vi "SPIM_LIVE.vi"() -> ()   [LabVIEW 2012]
panel:
  in  "Frames":i32=100
  out "Frames Recorded":i32=100
  in  "DCIMG Path":path=path "H:/test3.ps"
  out "Display":T1(plugin-control)
  out "Camera Serial":string="S/N: 730852"
  out "Camera Version":string="2.50.A"
  out "Camera Model":string="C11440-22C"
  out "SMD":dbl=2.0
  in  "Scan Mode":dbl=2.0 min=1.0 max=2.0 step=1.0
  in  "Exposure":dbl=0.00999771 min=0.0010036691729323308 max=10.0 step=1e-08
  out "EXP":dbl=0.00999771
  out "SVW":i32=2048
  out "SHW":i32=2048
  out "SVO":i32
  out "SHO":i32
  in  "V Width":i32=2048 min=1 max=512 step=1
  in  "V Offset":i32 min=0 max=0 step=1
  in  "H Width":i32=2048 min=1 max=512 step=1
  in  "H Offset":i32 min=0 max=0 step=1
  in  "Binning":u16(ring)=4 items=["1x1"=1, "2x2"=2, "4x4"=4]
  out "Elapsed Time":u32=7532
  out "Total Frames":i32=633
  in  "Display":bool=TRUE
  out "Frames Per Second":dbl=100.0
  out "error out":errorcluster
  in  "stop":bool
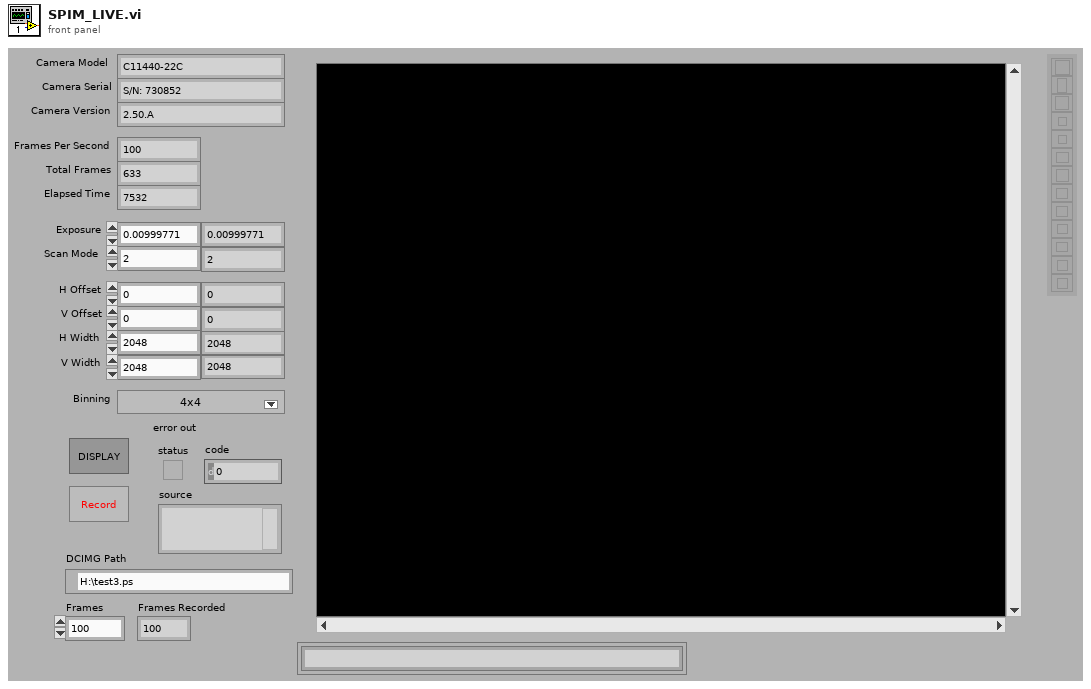
[diagram p1: front panel]
types:
  T1 = typedef "IMAQ Image.ctl" = refnum<image>
  T2 = typedef "Image Type" = u32
  T3 = cluster{"Value":i32, "Minimum":i32, "Maximum":i32, "Increment":i32}
  T4 = cluster{"width":u32, "height":u32, "datatype":u32}
  T5 = cluster{"H Offset":i32, "V Offset":i32, "H Width":i32, "V Width":i32}
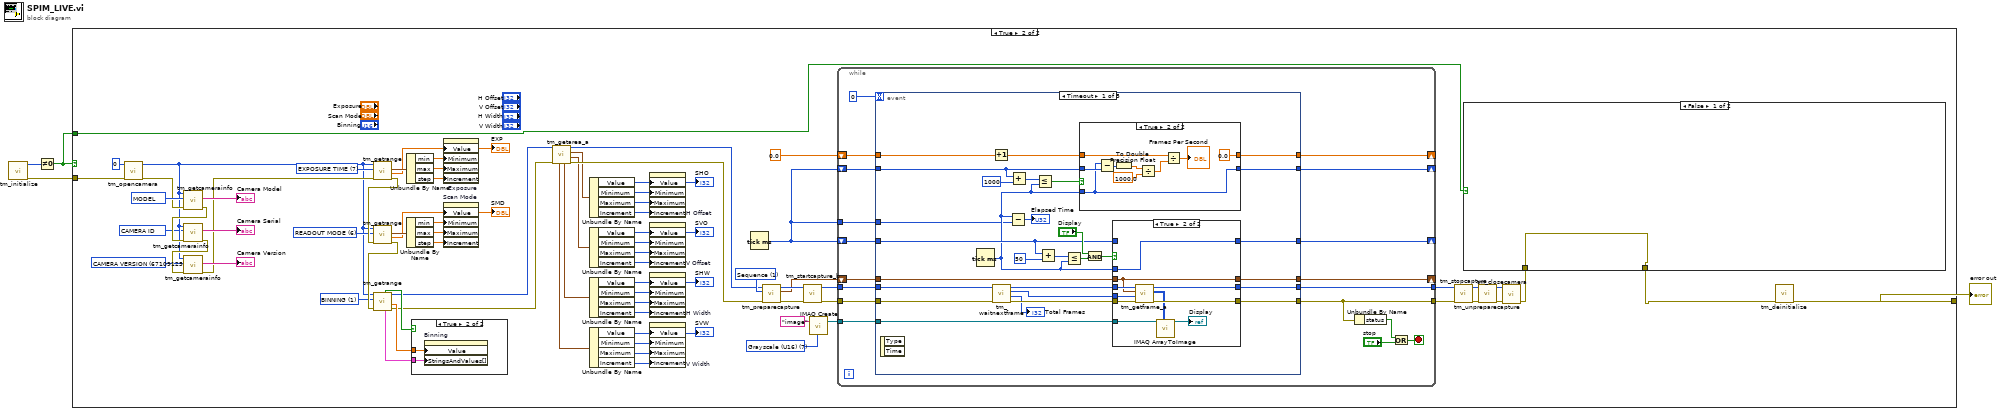
[diagram p0: block diagram]
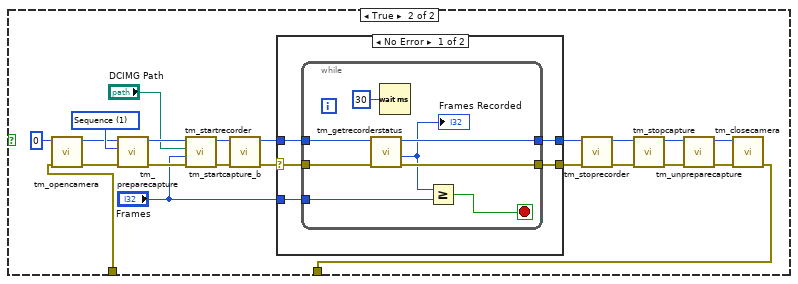
[diagram p3: hidden frame]
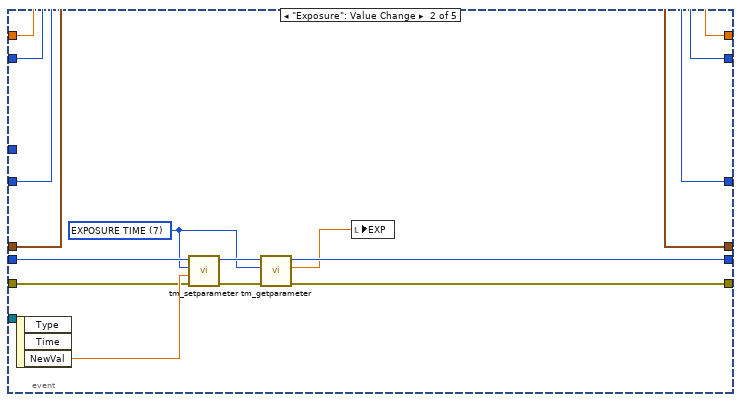
[diagram p8: hidden frame]
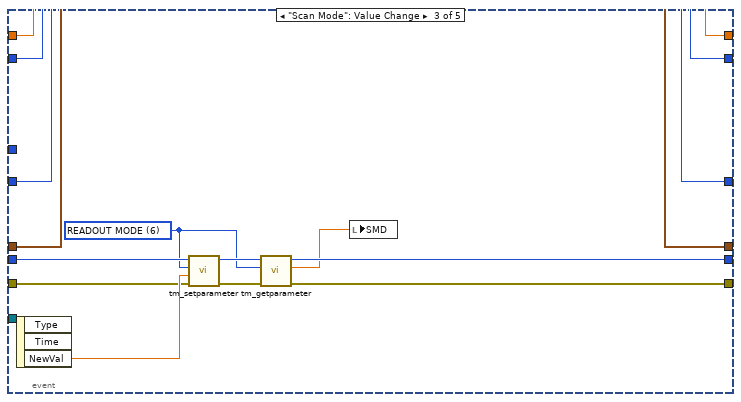
[diagram p9: hidden frame]
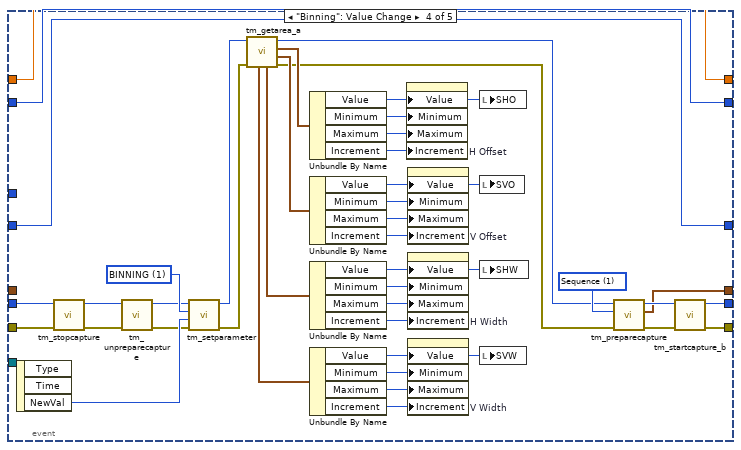
[diagram p10: hidden frame]
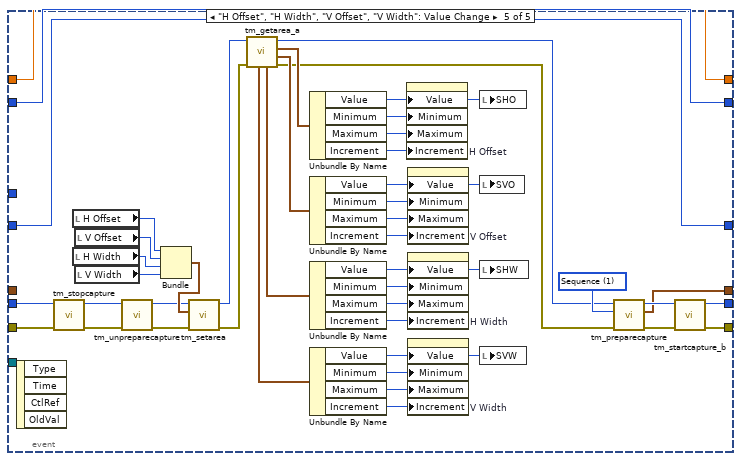
[diagram p11: hidden frame]
diagram:
  n1 = call <userlib>:"tm_initialize.vi"() -> ("error out"=w3:errorcluster, "Number Of Cameras"=w2:u32)  [unwired: 10 in]
  n2 = Not Equal To 0?(x=w2) -> (x != 0?=w1:bool)
  n3 = case shown="True" w1 {
    tunnel: [w5 w79] -> w4
    tunnel: w3 -> [w5 w81]
    tunnel: w1 -> [_ w8]
    frame False {
    }
    frame True {
      w9 = T2 7 items=["Grayscale (U8)", "Grayscale (I16)", "Grayscale (SGL)", "Complex (CSG)", "RGB (U32)", "HSL (U32)", "RGB (U64)", "Grayscale (U16)"] ("Image Type")
      w23 = u32 67109122 items=["BUS"=67109121, "CAMERA ID"=67109122, "VENDOR"=67109123, "MODEL"=67109124, "CAMERA VERSION"=67109125, "DRIVER VERSION"=67109126, "MODULE VERSIOIN"=67109127, "DCAMAPI VERSION"=67109128] ("Info ID")
      w30 = u32 67109125 items=["BUS"=67109121, "CAMERA"=67109122, "VENDOR"=67109123, "MODEL"=67109124, "CAMERA VERSION"=67109125, "DRIVER VERSION"=67109126, "MODULE VERSIOIN"=67109127, "DCAMAPI VERSION"=67109128] ("Info ID")
      w33 = u32 67109124 items=["BUS"=67109121, "CAMERA"=67109122, "VENDOR"=67109123, "MODEL"=67109124, "CAMERA VERSION"=67109125, "DRIVER VERSION"=67109126, "MODULE VERSIOIN"=67109127, "DCAMAPI VERSION"=67109128] ("Info ID")
      w65 = 1 items=["BINNING"=1, "BITS PER CHANNEL"=2, "ACTIVE VIEW INDEX"=3, "CCD MODE"=4, "SENSOR MODE"=5, "READOUT MODE"=6, "EXPOSURE TIME"=7, "CONTRAST GAIN"=8, "CONTRAST OFFSET"=9, "LIGHT MODE"=10, "SENSITIVITY"=11, "WHITE BALANCE"=12, "PHOTON IMAGING MODE"=13, "HIGH DYNAMIC RANGE MODE"=14, "TRIGGER SOURCE"=15, "TRIGGER ACTIVE"=16, "TRIGGER MODE"=17, "TRIGGER POLARITY"=18, "TRIGGER GLOBAL EXPOSURE"=19, "FIRST TRIGGER BEHAVIOR"=20, "TRIGGER TIMES"=21, "OUTPUT TRIGGER POLARITY"=22, "OUTPUT TRIGGER DELAY"=23, "OUTPUT TRIGGER PERIOD"=24, "TEMPERATURE"=25, "TEMPERATURE TARGET"=26, "SENSOR COOLER FAN"=27, "MECHANICAL SHUTTER"=28, "BACK FOCUS POSITION"=29, "FRAMEBUNDLE MODE"=30, "FRAMEBUNDLE NUMBER"=31] ("Parameter")
      w67 = 6 items=["BINNING"=1, "BITS PER CHANNEL"=2, "ACTIVE VIEW INDEX"=3, "CCD MODE"=4, "SENSOR MODE"=5, "READOUT MODE"=6, "EXPOSURE TIME"=7, "CONTRAST GAIN"=8, "CONTRAST OFFSET"=9, "LIGHT MODE"=10, "SENSITIVITY"=11, "WHITE BALANCE"=12, "PHOTON IMAGING MODE"=13, "HIGH DYNAMIC RANGE MODE"=14, "TRIGGER SOURCE"=15, "TRIGGER ACTIVE"=16, "TRIGGER MODE"=17, "TRIGGER POLARITY"=18, "TRIGGER GLOBAL EXPOSURE"=19, "FIRST TRIGGER BEHAVIOR"=20, "TRIGGER TIMES"=21, "OUTPUT TRIGGER POLARITY"=22, "OUTPUT TRIGGER DELAY"=23, "OUTPUT TRIGGER PERIOD"=24, "TEMPERATURE"=25, "TEMPERATURE TARGET"=26, "SENSOR COOLER FAN"=27, "MECHANICAL SHUTTER"=28, "BACK FOCUS POSITION"=29, "FRAMEBUNDLE MODE"=30, "FRAMEBUNDLE NUMBER"=31] ("Parameter")
      w70 = 7 items=["BINNING"=1, "BITS PER CHANNEL"=2, "ACTIVE VIEW INDEX"=3, "CCD MODE"=4, "SENSOR MODE"=5, "READOUT MODE"=6, "EXPOSURE TIME"=7, "CONTRAST GAIN"=8, "CONTRAST OFFSET"=9, "LIGHT MODE"=10, "SENSITIVITY"=11, "WHITE BALANCE"=12, "PHOTON IMAGING MODE"=13, "HIGH DYNAMIC RANGE MODE"=14, "TRIGGER SOURCE"=15, "TRIGGER ACTIVE"=16, "TRIGGER MODE"=17, "TRIGGER POLARITY"=18, "TRIGGER GLOBAL EXPOSURE"=19, "FIRST TRIGGER BEHAVIOR"=20, "TRIGGER TIMES"=21, "OUTPUT TRIGGER POLARITY"=22, "OUTPUT TRIGGER DELAY"=23, "OUTPUT TRIGGER PERIOD"=24, "TEMPERATURE"=25, "TEMPERATURE TARGET"=26, "SENSOR COOLER FAN"=27, "MECHANICAL SHUTTER"=28, "BACK FOCUS POSITION"=29, "FRAMEBUNDLE MODE"=30, "FRAMEBUNDLE NUMBER"=31] ("Parameter")
      w77 = 1 items=["Snap", "Sequence"] ("Capture mode")
      n4 = call <userlib>:"tm_opencamera.vi"("error in (no error)"=w81, "Camera Index"=u32 0) -> ("error out"=w26:errorcluster, "Handle out"=w24:u32)  [unwired: 8 in]
      n5 = call <userlib>:"tm_getcamerainfo.vi"("error in (no error)"=w26, "Info ID"=w33, "Handle in"=w24) -> ("error out"=w32:errorcluster, "String"=→"Camera Model":string)  [unwired: 6 in, 1 out]
      n6 = call <userlib>:"tm_getcamerainfo.vi"("error in (no error)"=w32, "Info ID"=w23, "Handle in"=w24) -> ("error out"=w31:errorcluster, "String"=→"Camera Serial":string)  [unwired: 6 in, 1 out]
      n7 = call <userlib>:"tm_getcamerainfo.vi"("error in (no error)"=w31, "Info ID"=w30, "Handle in"=w24) -> ("error out"=w25:errorcluster, "String"=→"Camera Version":string)  [unwired: 6 in, 1 out]
      n8 = call <userlib>:"tm_getrange.vi"("error in (no error)"=w25, "Parameter"=w70, "Handle in"=w24) -> ("error out"=w68:errorcluster, "default"=w61:dbl, "Range"=w69:cluster{"min":dbl, "max":dbl, "step":dbl})  [unwired: 2 in, 4 out]
      "EXP" <- w61
      n9 = call <userlib>:"tm_getrange.vi"("error in (no error)"=w68, "Parameter"=w67, "Handle in"=w24) -> ("error out"=w66:errorcluster, "default"=w56:dbl, "Range"=w60:cluster{"min":dbl, "max":dbl, "step":dbl})  [unwired: 2 in, 4 out]
      "SMD" <- w56
      n10 = call <userlib>:"tm_getrange.vi"("error in (no error)"=w66, "Parameter"=w65, "Handle in"=w24) -> ("error out"=w51:errorcluster, "default"=w53:dbl, "Handle out"=w52:u32, "Value Names"=w54:cluster{"Name":string, "Value":dbl}[], "Writable"=w55:bool)  [unwired: 2 in, 2 out]
      n11 = Unbundle By Name(w69) -> ("min"=w64:dbl, "max"=w63:dbl, "step"=w62:dbl)
      n12 = Unbundle By Name(w60) -> ("min"=w59:dbl, "max"=w58:dbl, "step"=w57:dbl)
      n13 = case shown="True" w55 {
        tunnel: w54 -> [_ w121]
        tunnel: w53 -> [_ w120]
        frame False {
        }
        frame True {
          n14 = property on="Binning" class="Ring (strict)"("Value"=w120, "StringsAndValues[]"=w121) -> ()  [unwired: 2 in, 2 out]
        }
      }
      n15 = property on="Exposure" class="DigNum (strict)"("Value"=w61, "Minimum"=w64, "Maximum"=w63, "Increment"=w62) -> ()  [unwired: 2 in, 2 out]
      n16 = property on="Scan Mode" class="DigNum (strict)"("Value"=w56, "Minimum"=w59, "Maximum"=w58, "Increment"=w57) -> ()  [unwired: 2 in, 2 out]
      n17 = call <userlib>:"tm_getarea_a.vi"("error in (no error)"=w51, "Handle in"=w52) -> ("error out"=w49:errorcluster, "V Offset"=w48:T3, "H Offset"=w16:T3, "Handle out"=w50:u32, "H Width"=w47:T3, "V Width"=w46:T3)  [unwired: 4 in]
      n18 = Unbundle By Name(w16) -> ("Value"=w15:i32, "Minimum"=w14:i32, "Maximum"=w13:i32, "Increment"=w12:i32)
      "SHO" <- w15
      n19 = Unbundle By Name(w48) -> ("Value"=w36:i32, "Minimum"=w45:i32, "Maximum"=w44:i32, "Increment"=w43:i32)
      "SVO" <- w36
      n20 = Unbundle By Name(w47) -> ("Value"=w35:i32, "Minimum"=w42:i32, "Maximum"=w41:i32, "Increment"=w40:i32)
      "SHW" <- w35
      n21 = Unbundle By Name(w46) -> ("Value"=w34:i32, "Minimum"=w39:i32, "Maximum"=w38:i32, "Increment"=w37:i32)
      "SVW" <- w34
      n22 = property on="H Offset" class="DigNum (strict)"("Value"=w15, "Minimum"=w14, "Maximum"=w13, "Increment"=w12) -> ()  [unwired: 2 in, 2 out]
      n23 = property on="V Offset" class="DigNum (strict)"("Value"=w36, "Minimum"=w45, "Maximum"=w44, "Increment"=w43) -> ()  [unwired: 2 in, 2 out]
      n24 = property on="H Width" class="DigNum (strict)"("Value"=w35, "Minimum"=w42, "Maximum"=w41, "Increment"=w40) -> ()  [unwired: 2 in, 2 out]
      n25 = property on="V Width" class="DigNum (strict)"("Value"=w34, "Minimum"=w39, "Maximum"=w38, "Increment"=w37) -> ()  [unwired: 2 in, 2 out]
      n26 = Tick Count (ms)() -> (millisecond timer value=w71:u32)
      n27 = call <userlib>:"tm_preparecapture.vi"("error in (no error)"=w49, "Capture mode"=w77, "Handle in"=w50) -> ("error out"=w75:errorcluster, "Buffer"=w72:T4, "Handle out"=w76:u32)  [unwired: 5 in, 1 out]
      n28 = call <userlib>:"tm_startcapture_b.vi"("error in (no error)"=w75, "Handle in"=w76) -> ("error out"=w74:errorcluster, "Handle out"=w73:u32)  [unwired: 8 in]
      n29 = call "IMAQ Create"("Image Name"="image", "Image Type"=w9) -> ("New Image"=w10:T1)  [unwired: 3 in, 1 out]
      n30 = while {
        tunnel: w74 -> [w127]
        tunnel: [w125] -> w22
        tunnel: [w124] -> w21
        shift-right: [w134] -> _
        shift-left: w71 -> [w132]
        shift-right: [w135] -> _
        shift-left: 0.0 -> [w133]
        shift-right: [w126] -> _
        shift-left: w71 -> [w130]
        tunnel: w73 -> [w128]
        tunnel: w71 -> [w131]
        shift-right: [w123] -> _
        shift-left: w72 -> [w129]
        tunnel: w10 -> [w122]
        stop <- w137 stop-if-true
        n31 = event shown="[0] Timeout" {
          selector: _ -> [_ _ _ _ _]
          dyn-events: _ -> [_ _ _ _ _]
          timeout: 0 -> [_ _ _ _ _]
          tunnel: [w148 w203 w216 w250 w296] -> w135
          tunnel: [w147 w204 w217 w251 w297] -> w134
          tunnel: w133 -> [w149 w203 w216 w250 w296]
          tunnel: w132 -> [w151 w204 w217 w251 w297]
          tunnel: w131 -> [w143 _ _ _ _]
          tunnel: w130 -> [w152 w206 w219 w260 w304]
          tunnel: w129 -> [w142 w195 w208 _ _]
          tunnel: w128 -> [w154 w201 w214 w225 w266]
          tunnel: w127 -> [w153 w202 w215 w224 w265]
          tunnel: [w146 w206 w219 w260 w304] -> w126
          tunnel: [w145 w197 w210 w254 w299] -> w125
          tunnel: [w144 w196 w209 w255 w300] -> w124
          tunnel: [w141 w195 w208 w253 w298] -> w123
          tunnel: w122 -> [w140 _ _ _ _]
          event Timeout {
            n32 = event-data() -> ()  [unwired: 1 in, 2 out]
            n33 = Tick Count (ms)() -> (millisecond timer value=w150:u32)
            n34 = Increment(x=w149) -> (x+1=w165:dbl)
            n35 = call <userlib>:"tm_waitnextframe.vi"("error in (no error)"=w153, "Handle in"=w154) -> ("error out"=w159:errorcluster, "Frame Count"=→"Total Frames":i32, "Frame Index"=w158:i32, "Handle out"=w160:u32)  [unwired: 6 in]
            n36 = Subtract(x=w150, y=w143) -> (x-y=→"Elapsed Time":u32)
            n37 = Add(x=w151, y=u32 1000) -> (x+y=w168:u32)
            n38 = Less Or Equal?(x=w168, y=w150) -> (x <= y?=w167:bool)
            n39 = Add(x=w152, y=u32 50) -> (x+y=w164:u32)
            n40 = Less Or Equal?(x=w164, y=w150) -> (x <= y?=w162:bool)
            n41 = case shown="True" w167 {
              tunnel: w151 -> [w184 w187]
              tunnel: [w184 w185] -> w147
              tunnel: w165 -> [w183 w191]
              tunnel: w150 -> [_ w185]
              tunnel: [w183 0.0] -> w148
              frame False {
              }
              frame True {
                n42 = Subtract(x=w185, y=w187) -> (x-y=w186:u32)
                n43 = To Double Precision Float(number=w186) -> (double precision float=w193:dbl)
                n44 = Divide(x=w193, y=1000.0) -> (x/y=w190:dbl)
                n45 = Divide(x=w191, y=w190) -> (x/y=→"Frames Per Second":dbl)
              }
            }
            n46 = And(x="Display", y=w162) -> (x .and. y?=w157:bool)
            n47 = case shown="True" w157 {
              tunnel: w152 -> [w172 _]
              tunnel: w150 -> [_ w182]
              tunnel: [w172 w182] -> w146
              tunnel: w160 -> [w171 w181]
              tunnel: w142 -> [w169 w176]
              tunnel: w159 -> [w170 w180]
              tunnel: [w171 w179] -> w145
              tunnel: [w170 w178] -> w144
              tunnel: w158 -> [_ w177]
              tunnel: [w169 w176] -> w141
              tunnel: w140 -> [_ w174]
              frame False {
              }
              frame True {
                n48 = call <userlib>:"tm_getframe_a.vi"("error in (no error)"=w180, "Frame Index"=w177, "Buffer"=w176, "Handle in"=w181) -> ("error out"=w178:errorcluster, "Data 16"=w175:u16[][], "Handle out"=w179:u32)  [unwired: 3 in, 2 out]
                n49 = call "IMAQ ArrayToImage"("Image Pixels (U16)"=w175, "Image"=w174) -> ("Image Out"=→"Display":T1)  [unwired: 8 in, 1 out]
              }
            }
          }
          event "Exposure": Value Change {
            w198 = 7 items=["BINNING"=1, "BITS PER CHANNEL"=2, "ACTIVE VIEW INDEX"=3, "CCD MODE"=4, "SENSOR MODE"=5, "READOUT MODE"=6, "EXPOSURE TIME"=7, "CONTRAST GAIN"=8, "CONTRAST OFFSET"=9, "LIGHT MODE"=10, "SENSITIVITY"=11, "WHITE BALANCE"=12, "PHOTON IMAGING MODE"=13, "HIGH DYNAMIC RANGE MODE"=14, "TRIGGER SOURCE"=15, "TRIGGER ACTIVE"=16, "TRIGGER MODE"=17, "TRIGGER POLARITY"=18, "TRIGGER GLOBAL EXPOSURE"=19, "FIRST TRIGGER BEHAVIOR"=20, "TRIGGER TIMES"=21, "OUTPUT TRIGGER POLARITY"=22, "OUTPUT TRIGGER DELAY"=23, "OUTPUT TRIGGER PERIOD"=24, "TEMPERATURE"=25, "TEMPERATURE TARGET"=26, "SENSOR COOLER FAN"=27, "MECHANICAL SHUTTER"=28, "BACK FOCUS POSITION"=29, "FRAMEBUNDLE MODE"=30, "FRAMEBUNDLE NUMBER"=31] ("Parameter")
            n50 = event-data() -> ("NewVal"=w205:dbl)  [unwired: 1 in, 2 out]
            n51 = call <userlib>:"tm_setparameter.vi"("error in (no error)"=w202, "Value in"=w205, "Parameter"=w198, "Handle in"=w201) -> ("error out"=w200:errorcluster, "Handle out"=w199:u32)  [unwired: 6 in]
            n52 = call <userlib>:"tm_getparameter.vi"("error in (no error)"=w200, "Parameter"=w198, "Handle in"=w199) -> ("error out"=w196:errorcluster, "Value out"=w194:dbl, "Handle out"=w197:u32)  [unwired: 6 in]
            n53 = local write "EXP"(w194) -> ()
          }
          event "Scan Mode": Value Change {
            w211 = 6 items=["BINNING"=1, "BITS PER CHANNEL"=2, "ACTIVE VIEW INDEX"=3, "CCD MODE"=4, "SENSOR MODE"=5, "READOUT MODE"=6, "EXPOSURE TIME"=7, "CONTRAST GAIN"=8, "CONTRAST OFFSET"=9, "LIGHT MODE"=10, "SENSITIVITY"=11, "WHITE BALANCE"=12, "PHOTON IMAGING MODE"=13, "HIGH DYNAMIC RANGE MODE"=14, "TRIGGER SOURCE"=15, "TRIGGER ACTIVE"=16, "TRIGGER MODE"=17, "TRIGGER POLARITY"=18, "TRIGGER GLOBAL EXPOSURE"=19, "FIRST TRIGGER BEHAVIOR"=20, "TRIGGER TIMES"=21, "OUTPUT TRIGGER POLARITY"=22, "OUTPUT TRIGGER DELAY"=23, "OUTPUT TRIGGER PERIOD"=24, "TEMPERATURE"=25, "TEMPERATURE TARGET"=26, "SENSOR COOLER FAN"=27, "MECHANICAL SHUTTER"=28, "BACK FOCUS POSITION"=29, "FRAMEBUNDLE MODE"=30, "FRAMEBUNDLE NUMBER"=31] ("Parameter")
            n54 = event-data() -> ("NewVal"=w218:dbl)  [unwired: 1 in, 2 out]
            n55 = call <userlib>:"tm_setparameter.vi"("error in (no error)"=w215, "Value in"=w218, "Parameter"=w211, "Handle in"=w214) -> ("error out"=w213:errorcluster, "Handle out"=w212:u32)  [unwired: 6 in]
            n56 = call <userlib>:"tm_getparameter.vi"("error in (no error)"=w213, "Parameter"=w211, "Handle in"=w212) -> ("error out"=w209:errorcluster, "Value out"=w207:dbl, "Handle out"=w210:u32)  [unwired: 6 in]
            n57 = local write "SMD"(w207) -> ()
          }
          event "Binning": Value Change {
            w258 = 1 items=["Snap", "Sequence"] ("Capture mode")
            w259 = 1 items=["BINNING"=1, "BITS PER CHANNEL"=2, "ACTIVE VIEW INDEX"=3, "CCD MODE"=4, "SENSOR MODE"=5, "READOUT MODE"=6, "EXPOSURE TIME"=7, "CONTRAST GAIN"=8, "CONTRAST OFFSET"=9, "LIGHT MODE"=10, "SENSITIVITY"=11, "WHITE BALANCE"=12, "PHOTON IMAGING MODE"=13, "HIGH DYNAMIC RANGE MODE"=14, "TRIGGER SOURCE"=15, "TRIGGER ACTIVE"=16, "TRIGGER MODE"=17, "TRIGGER POLARITY"=18, "TRIGGER GLOBAL EXPOSURE"=19, "FIRST TRIGGER BEHAVIOR"=20, "TRIGGER TIMES"=21, "OUTPUT TRIGGER POLARITY"=22, "OUTPUT TRIGGER DELAY"=23, "OUTPUT TRIGGER PERIOD"=24, "TEMPERATURE"=25, "TEMPERATURE TARGET"=26, "SENSOR COOLER FAN"=27, "MECHANICAL SHUTTER"=28, "BACK FOCUS POSITION"=29, "FRAMEBUNDLE MODE"=30, "FRAMEBUNDLE NUMBER"=31] ("Parameter")
            n58 = event-data() -> ("NewVal"=w252:u16)  [unwired: 1 in, 2 out]
            n59 = call <userlib>:"tm_stopcapture.vi"("error in (no error)"=w224, "Handle in"=w225) -> ("error out"=w220:errorcluster, "Handle out"=w223:u32)  [unwired: 8 in]
            n60 = call <userlib>:"tm_unpreparecapture.vi"("error in (no error)"=w220, "Handle in"=w223) -> ("error out"=w221:errorcluster, "Handle out"=w222:u32)  [unwired: 8 in]
            n61 = call <userlib>:"tm_setparameter.vi"("error in (no error)"=w221, "Value in"=w252, "Parameter"=w259, "Handle in"=w222) -> ("error out"=w244:errorcluster, "Handle out"=w245:u32)  [unwired: 6 in]
            n62 = call <userlib>:"tm_getarea_a.vi"("error in (no error)"=w244, "Handle in"=w245) -> ("error out"=w243:errorcluster, "V Offset"=w247:T3, "H Offset"=w246:T3, "Handle out"=w242:u32, "H Width"=w248:T3, "V Width"=w249:T3)  [unwired: 4 in]
            n63 = Unbundle By Name(w246) -> ("Value"=w238:i32, "Minimum"=w241:i32, "Maximum"=w240:i32, "Increment"=w239:i32)
            n64 = Unbundle By Name(w247) -> ("Value"=w228:i32, "Minimum"=w237:i32, "Maximum"=w236:i32, "Increment"=w235:i32)
            n65 = Unbundle By Name(w248) -> ("Value"=w227:i32, "Minimum"=w234:i32, "Maximum"=w233:i32, "Increment"=w232:i32)
            n66 = Unbundle By Name(w249) -> ("Value"=w226:i32, "Minimum"=w231:i32, "Maximum"=w230:i32, "Increment"=w229:i32)
            n67 = property on="H Offset" class="DigNum (strict)"("Value"=w238, "Minimum"=w241, "Maximum"=w240, "Increment"=w239) -> ()  [unwired: 2 in, 2 out]
            n68 = property on="V Offset" class="DigNum (strict)"("Value"=w228, "Minimum"=w237, "Maximum"=w236, "Increment"=w235) -> ()  [unwired: 2 in, 2 out]
            n69 = property on="H Width" class="DigNum (strict)"("Value"=w227, "Minimum"=w234, "Maximum"=w233, "Increment"=w232) -> ()  [unwired: 2 in, 2 out]
            n70 = property on="V Width" class="DigNum (strict)"("Value"=w226, "Minimum"=w231, "Maximum"=w230, "Increment"=w229) -> ()  [unwired: 2 in, 2 out]
            n71 = local write "SHO"(w238) -> ()
            n72 = local write "SVO"(w228) -> ()
            n73 = local write "SHW"(w227) -> ()
            n74 = local write "SVW"(w226) -> ()
            n75 = call <userlib>:"tm_preparecapture.vi"("error in (no error)"=w243, "Capture mode"=w258, "Handle in"=w242) -> ("error out"=w256:errorcluster, "Buffer"=w253:T4, "Handle out"=w257:u32)  [unwired: 5 in, 1 out]
            n76 = call <userlib>:"tm_startcapture_b.vi"("error in (no error)"=w256, "Handle in"=w257) -> ("error out"=w255:errorcluster, "Handle out"=w254:u32)  [unwired: 8 in]
          }
          event "H Offset", "H Width", "V Offset", "V Width": Value Change {
            w303 = 1 items=["Snap", "Sequence"] ("Capture mode")
            n77 = event-data() -> ()  [unwired: 1 in, 4 out]
            n78 = call <userlib>:"tm_stopcapture.vi"("error in (no error)"=w265, "Handle in"=w266) -> ("error out"=w263:errorcluster, "Handle out"=w264:u32)  [unwired: 8 in]
            n79 = local read "H Offset"() -> (w269:i32)
            n80 = local read "H Width"() -> (w270:i32)
            n81 = local read "V Offset"() -> (w271:i32)
            n82 = local read "V Width"() -> (w268:i32)
            n83 = call <userlib>:"tm_unpreparecapture.vi"("error in (no error)"=w263, "Handle in"=w264) -> ("error out"=w261:errorcluster, "Handle out"=w262:u32)  [unwired: 8 in]
            n84 = Bundle("H Offset"=w269, "V Offset"=w271, "H Width"=w270, "V Width"=w268) -> (w267:T5)  [unwired: 1 in]
            n85 = call <userlib>:"tm_setarea.vi"("error in (no error)"=w261, "Sub Region"=w267, "Handle in"=w262) -> ("error out"=w272:errorcluster, "Handle out"=w273:u32)  [unwired: 7 in]
            n86 = call <userlib>:"tm_getarea_a.vi"("error in (no error)"=w272, "Handle in"=w273) -> ("error out"=w291:errorcluster, "V Offset"=w293:T3, "H Offset"=w292:T3, "Handle out"=w290:u32, "H Width"=w294:T3, "V Width"=w295:T3)  [unwired: 4 in]
            n87 = Unbundle By Name(w292) -> ("Value"=w286:i32, "Minimum"=w289:i32, "Maximum"=w288:i32, "Increment"=w287:i32)
            n88 = Unbundle By Name(w293) -> ("Value"=w276:i32, "Minimum"=w285:i32, "Maximum"=w284:i32, "Increment"=w283:i32)
            n89 = Unbundle By Name(w294) -> ("Value"=w275:i32, "Minimum"=w282:i32, "Maximum"=w281:i32, "Increment"=w280:i32)
            n90 = Unbundle By Name(w295) -> ("Value"=w274:i32, "Minimum"=w279:i32, "Maximum"=w278:i32, "Increment"=w277:i32)
            n91 = property on="H Offset" class="DigNum (strict)"("Value"=w286, "Minimum"=w289, "Maximum"=w288, "Increment"=w287) -> ()  [unwired: 2 in, 2 out]
            n92 = property on="V Offset" class="DigNum (strict)"("Value"=w276, "Minimum"=w285, "Maximum"=w284, "Increment"=w283) -> ()  [unwired: 2 in, 2 out]
            n93 = property on="H Width" class="DigNum (strict)"("Value"=w275, "Minimum"=w282, "Maximum"=w281, "Increment"=w280) -> ()  [unwired: 2 in, 2 out]
            n94 = property on="V Width" class="DigNum (strict)"("Value"=w274, "Minimum"=w279, "Maximum"=w278, "Increment"=w277) -> ()  [unwired: 2 in, 2 out]
            n95 = local write "SHO"(w286) -> ()
            n96 = local write "SVO"(w276) -> ()
            n97 = local write "SHW"(w275) -> ()
            n98 = local write "SVW"(w274) -> ()
            n99 = call <userlib>:"tm_preparecapture.vi"("error in (no error)"=w291, "Capture mode"=w303, "Handle in"=w290) -> ("error out"=w301:errorcluster, "Buffer"=w298:T4, "Handle out"=w302:u32)  [unwired: 5 in, 1 out]
            n100 = call <userlib>:"tm_startcapture_b.vi"("error in (no error)"=w301, "Handle in"=w302) -> ("error out"=w300:errorcluster, "Handle out"=w299:u32)  [unwired: 8 in]
          }
        }
        n101 = Unbundle By Name(w124) -> ("status"=w138:bool)
        n102 = Or(x=w138, y="stop") -> (x .or. y?=w137:bool)
      }
      n103 = call <userlib>:"tm_stopcapture.vi"("error in (no error)"=w21, "Handle in"=w22) -> ("error out"=w18:errorcluster, "Handle out"=w19:u32)  [unwired: 8 in]
      n104 = call <userlib>:"tm_unpreparecapture.vi"("error in (no error)"=w18, "Handle in"=w19) -> ("error out"=w17:errorcluster, "Handle out"=w20:u32)  [unwired: 8 in]
      n105 = call <userlib>:"tm_closecamera.vi"("error in (no error)"=w17, "Handle in"=w20) -> ("error out"=w7:errorcluster)  [unwired: 9 in]
      n106 = case shown="False" w8 {
        tunnel: w7 -> [w82 w84]
        tunnel: [w82 w83] -> w6
        frame False {
        }
        frame True {
          w103 = 1 items=["Snap", "Sequence"] ("Capture mode")
          n107 = call <userlib>:"tm_opencamera.vi"("error in (no error)"=w84, "Camera Index"=u32 0) -> ("error out"=w91:errorcluster, "Handle out"=w92:u32)  [unwired: 8 in]
          n108 = call <userlib>:"tm_preparecapture.vi"("error in (no error)"=w91, "Capture mode"=w103, "Handle in"=w92) -> ("error out"=w100:errorcluster, "Handle out"=w99:u32)  [unwired: 5 in, 2 out]
          n109 = call <userlib>:"tm_startrecorder.vi"("error in (no error)"=w100, "frames"="Frames", "File"="DCIMG Path", "Handle in"=w99) -> ("error out"=w98:errorcluster, "Handle out"=w97:u32)  [unwired: 6 in]
          n110 = call <userlib>:"tm_startcapture_b.vi"("error in (no error)"=w98, "Handle in"=w97) -> ("error out"=w96:errorcluster, "Handle out"=w95:u32)  [unwired: 8 in]
          n111 = case shown="No Error" w96 {
            selector: w96 -> [w109 w118]
            tunnel: w95 -> [w108 w119]
            tunnel: [w106 w119] -> w85
            tunnel: [w107 w118] -> w86
            tunnel: "Frames" -> [w105 _]
            frame No Error {
              n112 = while {
                tunnel: w109 -> [w115]
                tunnel: w108 -> [w114]
                tunnel: [w113] -> w107
                tunnel: [w116] -> w106
                tunnel: w105 -> [w117]
                stop <- w111 stop-if-true
                n113 = call <userlib>:"tm_getrecorderstatus.vi"("error in (no error)"=w115, "Handle"=w114) -> ("error out"=w113:errorcluster, "Count"=w112:i32, "Handle"=w116:u32)  [unwired: 6 in, 1 out]
                "Frames Recorded" <- w112
                n114 = Wait (ms)(milliseconds to wait=u32 30) -> ()  [unwired: 1 out]
                n115 = Greater Or Equal?(x=w112, y=w117) -> (x >= y?=w111:bool)
              }
            }
            frame Error {
            }
          }
          n116 = call <userlib>:"tm_stoprecorder.vi"("error in (no error)"=w86, "Handle in"=w85) -> ("error out"=w87:errorcluster, "Handle out"=w88:u32)  [unwired: 8 in]
          n117 = call <userlib>:"tm_stopcapture.vi"("error in (no error)"=w87, "Handle in"=w88) -> ("error out"=w90:errorcluster, "Handle out"=w89:u32)  [unwired: 8 in]
          n118 = call <userlib>:"tm_unpreparecapture.vi"("error in (no error)"=w90, "Handle in"=w89) -> ("error out"=w102:errorcluster, "Handle out"=w101:u32)  [unwired: 8 in]
          n119 = call <userlib>:"tm_closecamera.vi"("error in (no error)"=w102, "Handle in"=w101) -> ("error out"=w83:errorcluster)  [unwired: 9 in]
        }
      }
      n120 = call <userlib>:"tm_deinitialize.vi"("error in (no error)"=w6) -> ("error out"=w79:errorcluster)  [unwired: 10 in]
    }
  }
  "error out" <- w4
